vi "Init.vi"(8 "error in (no error)":errorcluster, 10 "Initial Setting":variant, 11 "Abstract Instrument in":refnum<class "Abstract Instrument.lvclass">) -> (0 "error out":errorcluster, 2 "Found?":bool=TRUE, 3 "Abstract Instrument out":refnum<class "Abstract Instrument.lvclass">)   [LabVIEW 2025, in "Abstract Engine.lvlib" / "Abstract Instrument.lvclass"]
uses:
  Abstract Instrument.lvclass
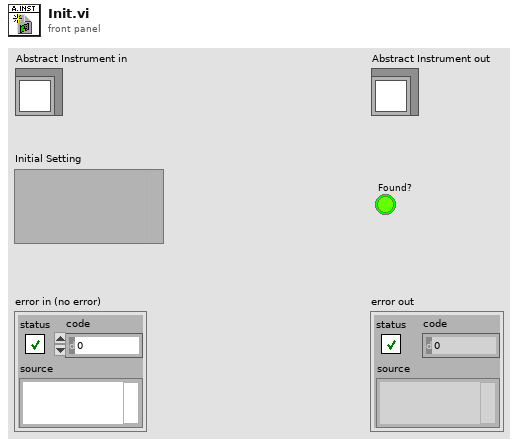
[diagram p1: front panel]
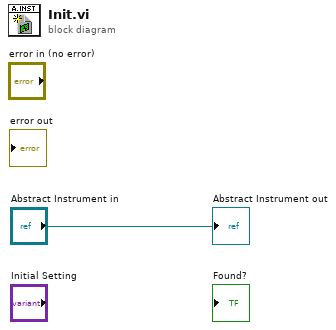
[diagram p0: block diagram]
diagram:
  "Abstract Instrument out" <- "Abstract Instrument in"
